vi "Average Done.vi"(11 "Imaging data processed":u32) -> (2 "Imaging data address":u32, 3 "Average Done":bool)   [LabVIEW 2015]
uses:
  Globals/Global_Sample per Frame.vi
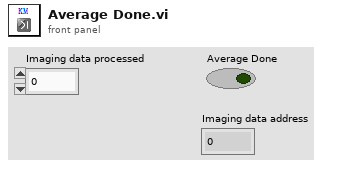
[diagram p1: front panel]
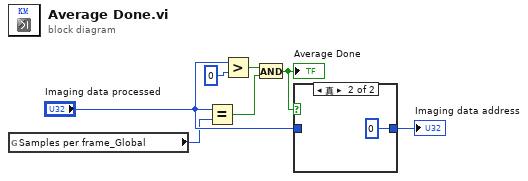
[diagram p0: block diagram]
diagram:
  n1 = global read "Global_Sample per Frame.vi" "Samples per frame_Global"() -> (w4:u32)
  n2 = Equal?(x="Imaging data processed", y=w4) -> (x = y?=w3:bool)
  n3 = Greater?(x="Imaging data processed", y=u32 0) -> (0:w2:bool)
  n4 = And(x=w2, y=w3) -> (x .and. y?=w5:bool)
  "Average Done" <- w5
  n5 = case shown="真" w5 {
    tunnel: [w8 u32 0 ("Imaging data address")] -> w6
    tunnel: "Imaging data processed" -> [w8 _]
    frame False {
    }
    frame True {
    }
  }
  "Imaging data address" <- w6
